vi "Get Camera Target.vi"(11 "Track Ball?":bool) -> (1 "Camera Relative Y":dbl, 2 "Found?":bool, 3 "Camera Relative X":dbl)   [LabVIEW 2013]
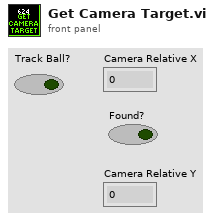
[diagram p1: front panel]
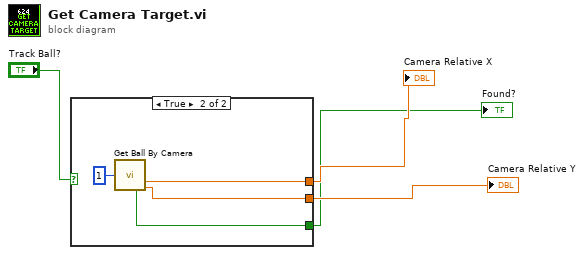
[diagram p0: block diagram]
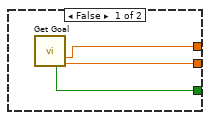
[diagram p2: hidden frame]
diagram:
  n1 = case shown="True" "Track Ball?" {
    tunnel: [w7 w11] -> w4
    tunnel: [w6 w10] -> w2
    tunnel: [w5 w9] -> w3
    frame False {
      n2 = call "Get Goal.vi"() -> ("Camera Relative X (Target)"=w7:dbl, "Goal Found?"=w6:bool, "Camera Relative Y (Target)"=w5:dbl)  [unwired: 7 in, 6 out]
    }
    frame True {
      n3 = call "Get Ball By Camera.vi"("Camera"=i16 1) -> ("Camera Relative X"=w11:dbl, "Ball Found?"=w10:bool, "Camera Relative Y"=w9:dbl)  [unwired: 9 in, 3 out]
    }
  }
  "Camera Relative X" <- w4
  "Camera Relative Y" <- w3
  "Found?" <- w2
